vi "Get_Joystick.vi"(1 "Joystick_One":string="Pilot Controller", 2 "Joystick_Two":string="CoPilot Controller") -> (6 "Joystick_Out":T1)   [LabVIEW 2018]
uses:
  Joystick_Controls.ctl
  <vilib>/Rock Robotics/WPI/Utilities/WPI_GetSetVariantRefNum.vi
panel:
  in  "Joystick Controls":T1
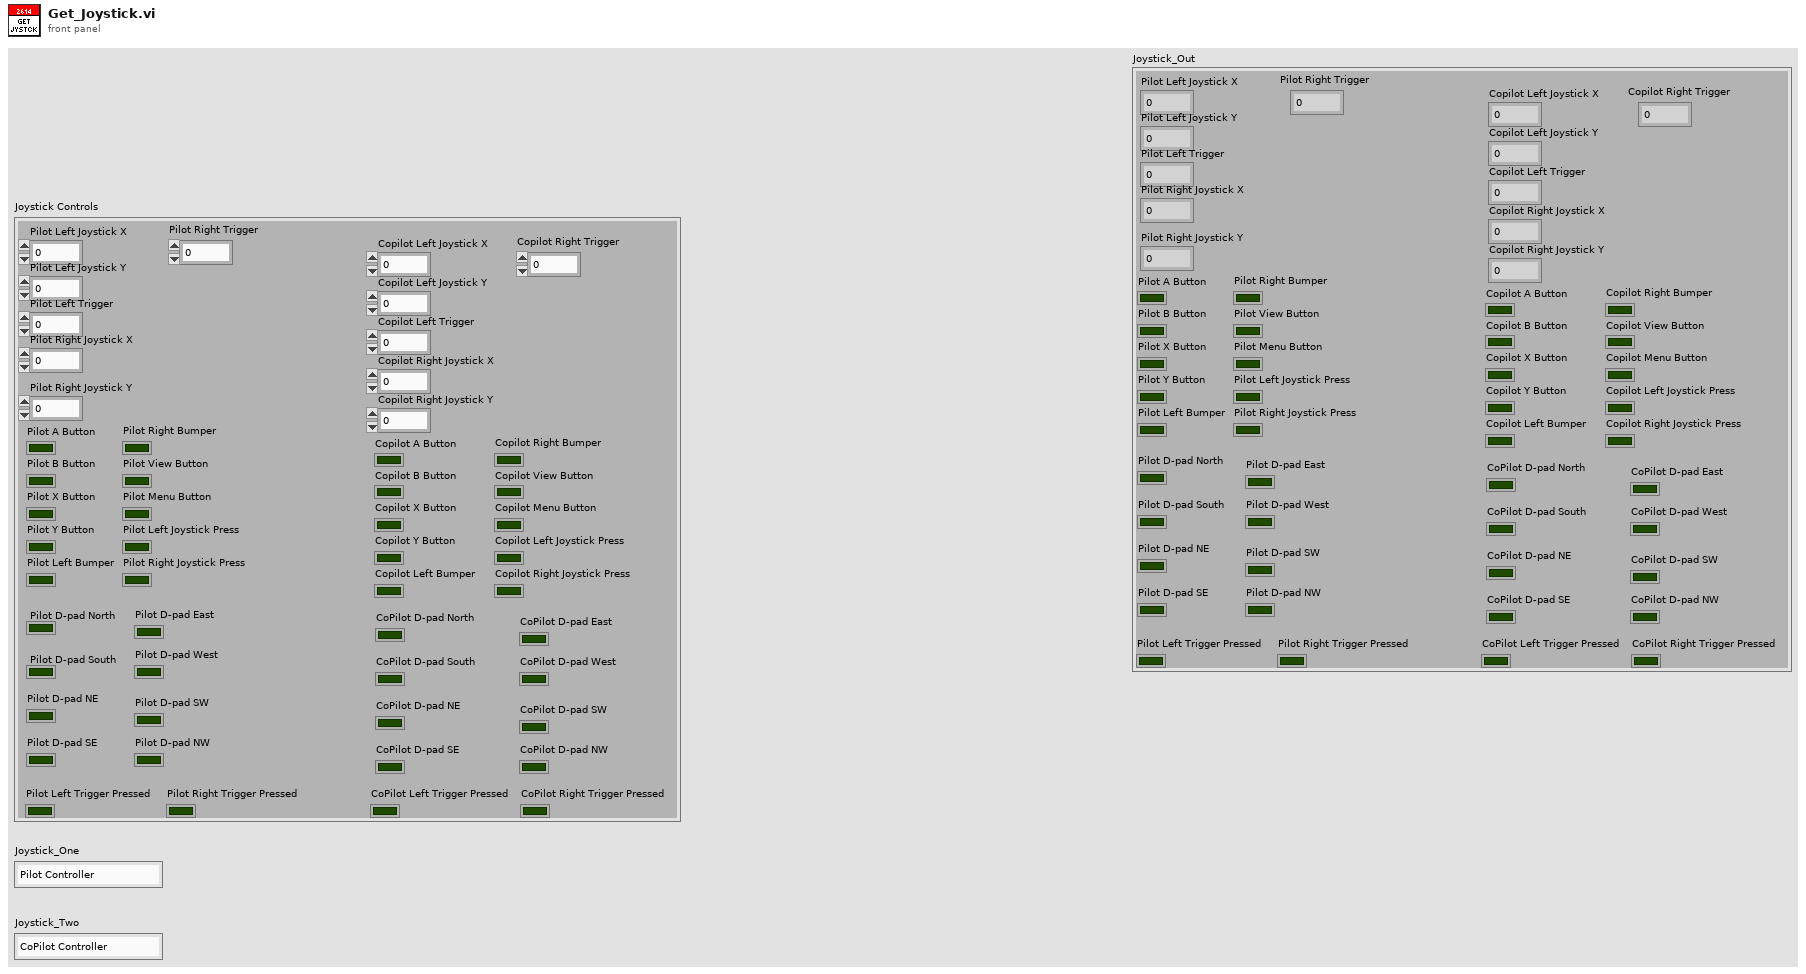
[diagram p1: front panel]
types:
  T1 = typedef "Joystick_Controls.ctl" = cluster{"Pilot Left Joystick X":dbl, "Pilot Left Joystick Y":dbl, "Pilot A Button":bool, "Pilot B Button":bool, "Pilot X Button":bool, "Pilot Y Button":bool, "Pilot Left Bumper":bool, "Pilot Right Bumper":bool, "Pilot View Button":bool, "Pilot Menu Button":bool, "Pilot Left Joystick Press":bool, "Pilot Right Joystick Press":bool, "Pilot Left Trigger":dbl, "Pilot Right Joystick X":dbl, "Pilot Right Joystick Y":dbl, "Pilot Right Trigger":dbl, "Copilot Left Joystick X":dbl, "Copilot Left Joystick Y":dbl, "Copilot A Button":bool, "Copilot B Button":bool, "Copilot X Button":bool, "Copilot Y Button":bool, "Copilot Left Bumper":bool, "Copilot Right Bumper":bool, "Copilot View Button":bool, "Copilot Menu Button":bool, "Copilot Left Joystick Press":bool, "Copilot Right Joystick Press":bool, "Copilot Left Trigger":dbl, "Copilot Right Joystick X":dbl, "Copilot Right Joystick Y":dbl, "Copilot Right Trigger":dbl, "Pilot D-pad North":bool, "Pilot D-pad South":bool, "Pilot D-pad East":bool, "Pilot D-pad West":bool, "Pilot D-pad NE ":bool, "Pilot D-pad SE":bool, "Pilot D-pad SW":bool, "Pilot D-pad NW":bool, "CoPilot D-pad North":bool, "CoPilot D-pad South":bool, "CoPilot D-pad East":bool, "CoPilot D-pad West":bool, "CoPilot D-pad NE":bool, "CoPilot D-pad SE":bool, "CoPilot D-pad SW":bool, "CoPilot D-pad NW":bool, "Pilot Left Trigger Pressed":bool, "Pilot Right Trigger Pressed":bool, "CoPilot Left Trigger Pressed":bool, "CoPilot Right Trigger Pressed":bool}
  T2 = typedef "WPI_JoystickDevRef.ctl" = cluster{"Device":T3}
  T3 = typedef "WPI_JoystickDeviceEnum.ctl" = enum16{"USB 0", "USB 1", "USB 2", "USB 3", "USB 4", "USB 5"}
  T4 = cluster{"Axes[0]":dbl, "Axes[1]":dbl, "Axes[2]":dbl, "Axes[3]":dbl, "Axes[4]":dbl, "Axes[5]":dbl, "Axes[6]":dbl, "Axes[7]":dbl, "Axes[8]":dbl}
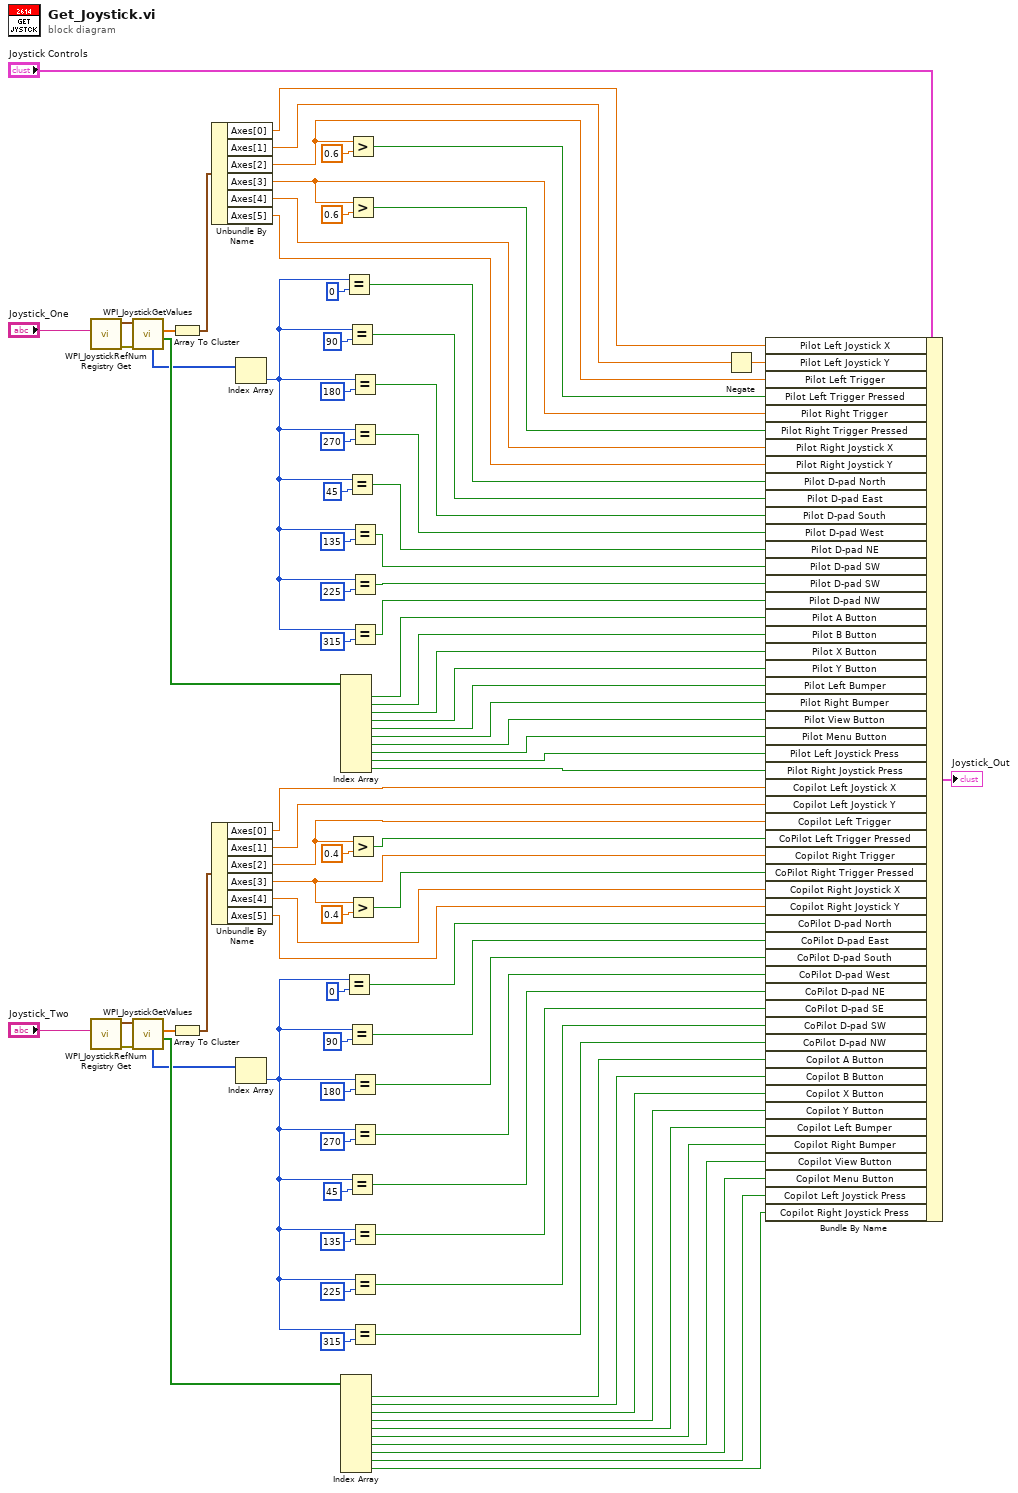
[diagram p0: block diagram]
diagram:
  n1 = call <vilib>:"WPI_JoystickRefNum Registry Get.vi"("refnum name"="Joystick_One") -> ("error out"=w52:errorcluster, "JoystickDevRef"=w91:T2)  [unwired: 9 in]
  n2 = call <vilib>:"WPI_JoystickRefNum Registry Get.vi"("refnum name"="Joystick_Two") -> ("error out"=w51:errorcluster, "JoystickDevRef"=w73:T2)  [unwired: 9 in]
  n3 = call <vilib>:"WPI_JoystickGetValues.vi"("error in (no error)"=w52, "JoystickDevRef"=w91) -> ("Buttons"=w84:bool[], "Axes"=w90:dbl[], "POVs"=w54:i16[])  [unwired: 5 in, 2 out]
  n4 = call <vilib>:"WPI_JoystickGetValues.vi"("error in (no error)"=w51, "JoystickDevRef"=w73) -> ("Buttons"=w71:bool[], "Axes"=w72:dbl[], "POVs"=w53:i16[])  [unwired: 5 in, 2 out]
  n5 = Array To Cluster(array=w90) -> (cluster=w89:T4)
  n6 = Array To Cluster(array=w72) -> (cluster=w70:T4)
  n7 = Unbundle By Name(w89) -> ("Axes[0]"=w88:dbl, "Axes[1]"=w87:dbl, "Axes[2]"=w15:dbl, "Axes[3]"=w11:dbl, "Axes[4]"=w86:dbl, "Axes[5]"=w85:dbl)
  n8 = Unbundle By Name(w70) -> ("Axes[0]"=w69:dbl, "Axes[1]"=w68:dbl, "Axes[2]"=w8:dbl, "Axes[3]"=w5:dbl, "Axes[4]"=w67:dbl, "Axes[5]"=w66:dbl)
  n9 = Index Array(array=w54) -> (element=w41:i16)  [unwired: 1 in]
  n10 = Index Array(array=w53) -> (element=w16:i16)  [unwired: 1 in]
  n11 = Index Array(array=w84) -> (element #1=w83:bool, element #2=w82:bool, element #3=w81:bool, element #4=w80:bool, element #5=w79:bool, element #6=w78:bool, element #7=w77:bool, element #8=w76:bool, element #9=w75:bool, element #10=w74:bool)  [unwired: 10 in]
  n12 = Index Array(array=w71) -> (element #1=w65:bool, element #2=w64:bool, element #3=w63:bool, element #4=w62:bool, element #5=w60:bool, element #6=w61:bool, element #7=w59:bool, element #8=w58:bool, element #9=w57:bool, element #10=w56:bool)  [unwired: 10 in]
  n13 = Equal?(x=w41, y=i16 0) -> (x = y?=w2:bool)
  n14 = Equal?(x=w16, y=i16 0) -> (x = y?=w24:bool)
  n15 = Equal?(x=w41, y=i16 90) -> (x = y?=w48:bool)
  n16 = Equal?(x=w41, y=i16 45) -> (x = y?=w44:bool)
  n17 = Equal?(x=w16, y=i16 90) -> (x = y?=w23:bool)
  n18 = Equal?(x=w16, y=i16 45) -> (x = y?=w20:bool)
  n19 = Greater?(x=w15, y=0.6) -> (0:w13:bool)
  n20 = Greater?(x=w11, y=0.6) -> (0:w12:bool)
  n21 = Greater?(x=w8, y=0.4) -> (0:w9:bool)
  n22 = Greater?(x=w5, y=0.4) -> (0:w6:bool)
  n23 = Equal?(x=w41, y=i16 180) -> (x = y?=w47:bool)
  n24 = Equal?(x=w41, y=i16 270) -> (x = y?=w46:bool)
  n25 = Equal?(x=w41, y=i16 135) -> (x = y?=w43:bool)
  n26 = Equal?(x=w41, y=i16 225) -> (x = y?=w42:bool)
  n27 = Equal?(x=w41, y=i16 315) -> (x = y?=w45:bool)
  n28 = Equal?(x=w16, y=i16 180) -> (x = y?=w22:bool)
  n29 = Equal?(x=w16, y=i16 270) -> (x = y?=w21:bool)
  n30 = Equal?(x=w16, y=i16 135) -> (x = y?=w19:bool)
  n31 = Equal?(x=w16, y=i16 225) -> (x = y?=w18:bool)
  n32 = Equal?(x=w16, y=i16 315) -> (x = y?=w17:bool)
  n33 = Negate(x=w87) -> (-x=w1:dbl)
  n34 = Bundle By Name(cluster="Joystick Controls", "Pilot Left Joystick X"=w88, "Pilot Left Joystick Y"=w1, "Pilot Left Trigger"=w15, "Pilot Left Trigger Pressed"=w13, "Pilot Right Trigger"=w11, "Pilot Right Trigger Pressed"=w12, "Pilot Right Joystick X"=w86, "Pilot Right Joystick Y"=w85, "Pilot D-pad North"=w2, "Pilot D-pad East"=w48, "Pilot D-pad South"=w47, "Pilot D-pad West"=w46, "Pilot D-pad NE"=w44, "Pilot D-pad SW"=w43, "Pilot D-pad SW"=w42, "Pilot D-pad NW"=w45, "Pilot A Button"=w83, "Pilot B Button"=w82, "Pilot X Button"=w81, "Pilot Y Button"=w80, "Pilot Left Bumper"=w79, "Pilot Right Bumper"=w78, "Pilot View Button"=w77, "Pilot Menu Button"=w76, "Pilot Left Joystick Press"=w75, "Pilot Right Joystick Press"=w74, "Copilot Left Joystick X"=w69, "Copilot Left Joystick Y"=w68, "Copilot Left Trigger"=w8, "CoPilot Left Trigger Pressed"=w9, "Copilot Right Trigger"=w5, "CoPilot Right Trigger Pressed"=w6, "Copilot Right Joystick X"=w67, "Copilot Right Joystick Y"=w66, "CoPilot D-pad North"=w24, "CoPilot D-pad East"=w23, "CoPilot D-pad South"=w22, "CoPilot D-pad West"=w21, "CoPilot D-pad NE"=w20, "CoPilot D-pad SE"=w19, "CoPilot D-pad SW"=w18, "CoPilot D-pad NW"=w17, "Copilot A Button"=w65, "Copilot B Button"=w64, "Copilot X Button"=w63, "Copilot Y Button"=w62, "Copilot Left Bumper"=w60, "Copilot Right Bumper"=w61, "Copilot View Button"=w59, "Copilot Menu Button"=w58, "Copilot Left Joystick Press"=w57, "Copilot Right Joystick Press"=w56) -> (→"Joystick_Out":T1)
